vi "test.vi"(8 "error in (no error)":errorcluster caption="エラー入力（エラーなし）", 10 "ブール":bool, 11 "child 入力":refnum<class "child.lvclass">) -> (0 "error out":errorcluster caption="エラー出力", 3 "child 出力":refnum<class "child.lvclass">)   [LabVIEW 2014, in "child.lvclass"]
uses:
  child.lvclass
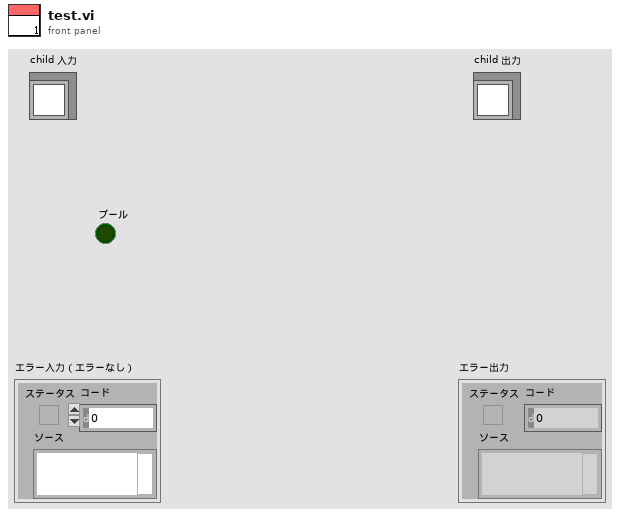
[diagram p1: front panel]
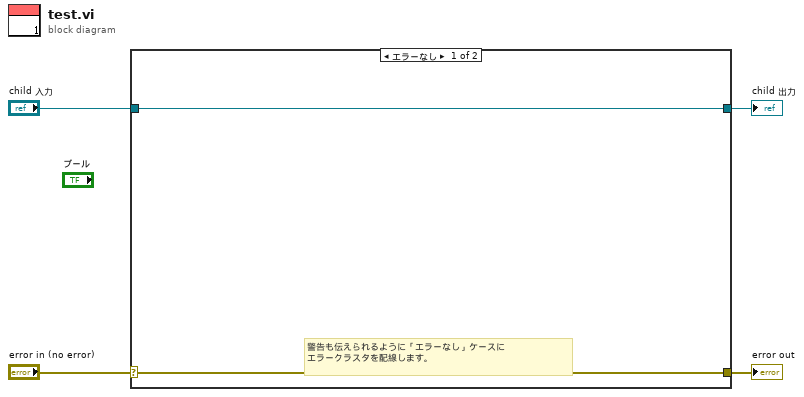
[diagram p0: block diagram]
diagram:
  n1 = case shown="エラーなし" "error in (no error)" {
    selector: "error in (no error)" -> [w5 w8]
    tunnel: [w5 w8] -> w3
    tunnel: [w6 w7] -> w1
    tunnel: "child 入力" -> [w6 w7]
    frame No Error {
      # "警告も伝えられるように「エラーなし」ケースに\nエラークラスタを配線します。"
    }
    frame Error {
    }
  }
  "error out" <- w3
  "child 出力" <- w1
